vi "LV Semaphore Open Acquire.vi"(7 "Timeout (ms)":i32=65535, 8 "error in":errorcluster, 11 "Name":string="LabVIEW_System_Semaphore") -> (0 "error out":errorcluster, 2 "Timed Out?":bool, 3 "semaphore":T1)   [LabVIEW 2011]
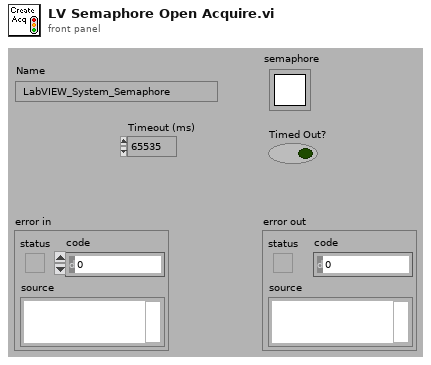
[diagram p1: front panel]
types:
  T1 = typedef "Semaphore RefNum" = refnum<k1>
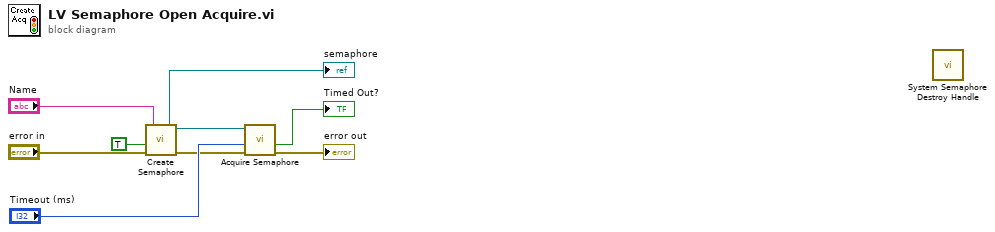
[diagram p0: block diagram]
diagram:
  n1 = call <vilib>:"Create Semaphore.vi"("error in (no error)"="error in", "return existing (F)"=TRUE, "name (unnamed)"="Name") -> ("error out"=w2:errorcluster, "semaphore"=w4:T1)  [unwired: 1 in, 2 out]
  "semaphore" <- w4
  n2 = call <vilib>:"Acquire Semaphore.vi"("error in (no error)"=w2, "ms timeout (-1)"="Timeout (ms)", "semaphore"=w4) -> ("error out"=→"error out":errorcluster, "timed out"=→"Timed Out?":bool)  [unwired: 3 out]
  n3 = call "System Semaphore Destroy Handle.vi"() -> ()  [unwired: 2 in, 10 out]
